vi "Absolute To Relative Path.vi"(0 "url in":string, 11 "error in (no error)":errorcluster) -> (4 "url out":string, 15 "error out":errorcluster)   [LabVIEW 2014, in "lvprj2html.lvlib"]
uses:
  lvprj2html.lvlib
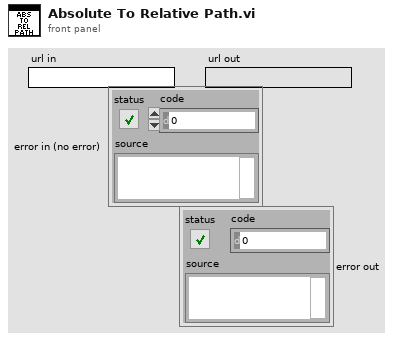
[diagram p1: front panel]
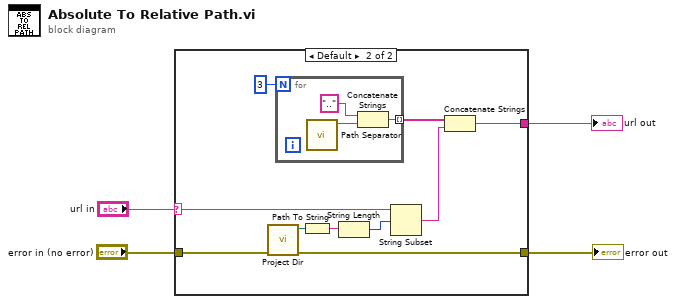
[diagram p0: block diagram]
diagram:
  n1 = case shown="Default" "url in" {
    selector: "url in" -> [w6 w7]
    tunnel: "error in (no error)" -> [w5 w13]
    tunnel: [w5 w12] -> w3
    tunnel: [w6 w8] -> w2
    frame "\u0000" {
    }
    frame Default {
      n2 = call "Project Dir.vi"("error in (no error)"=w13) -> ("error out"=w12:errorcluster, "path"=w14:path)  [unwired: 9 in]
      n3 = for {
        N: 3 -> [_]
        tunnel: [w17] -> w10 mode=indexing
        n4 = call "Path Separator.vi"() -> ("separator"=w18:string)  [unwired: 11 in]
        n5 = Concatenate Strings(".." ("string"), w18) -> (w17:string)
      }
      n6 = Path To String(path=w14) -> (string=w15:string)
      n7 = String Length(string=w15) -> (length=w16:i32)
      n8 = String Subset(string=w7, offset (0)=w16) -> (substring=w9:string)  [unwired: 1 in]
      n9 = Concatenate Strings(w10, w9) -> (w8:string)
    }
  }
  "url out" <- w2
  "error out" <- w3
